vi "Test.vi"() -> ()   [LabVIEW 2020]
panel:
  out "Reading":bool
  out "Connected":bool
  out "Numeric":dbl
  out "Text":string caption="Result"
  in  "stop":bool
  in  "COM Bluegiga in":refnum<visa-resource-name>="COM13"
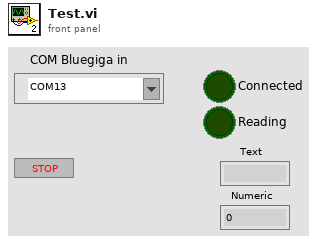
[diagram p1: front panel]
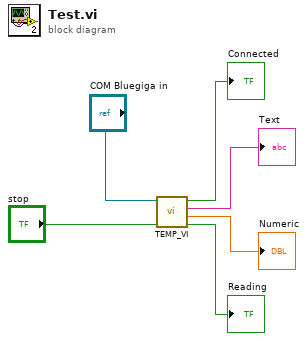
[diagram p0: block diagram]
diagram:
  n1 = call "TEMP_VI.vi"("stop"="stop", "COM Bluegiga in"="COM Bluegiga in") -> ("Reading"=→"Reading":bool, "Numeric"=→"Numeric":dbl, "Text"=→"Text":string, "Connected"=→"Connected":bool)  [unwired: 6 in]
